vi "Keysight 34401A Cancellation Logic.vi"(8 "error in (no error)":errorcluster, 9 "session information":T1, 10 "measurement complete":refnum<user-event>, 11 "MeasurementContext in":refnum<class "MeasurementContext.lvclass">) -> (0 "error out":errorcluster, 3 "MeasurementContext out":refnum<class "MeasurementContext.lvclass">)   [LabVIEW 2020, in "Keysight 34401A DMM Measurement.lvlib"]
uses:
  Keysight 34401A DMM Measurement.lvlib
  <instrlib>/Agilent 34401/Agilent 34401.lvlib
  <vilib>/MeasurementLink/MeasurementLink Session Management Client/RPC Messages/ni_measurementlink_sessionmanagement_v1_ChannelMapping.ctl
  <vilib>/MeasurementLink/MeasurementLink Session Management Client/MeasurementLink Session Management Client.lvlib
  <vilib>/MeasurementLink/MeasurementLink Session Management Client/RPC Messages/nidevice_grpc_Session.ctl
  <vilib>/MeasurementLink/MeasurementLink Session Management Client/RPC Messages/ni_measurementlink_sessionmanagement_v1_SessionInformation.ctl
  <vilib>/MeasurementLink/MeasurementLink Measurement Server/Classes/MeasurementContext/MeasurementContext.lvclass
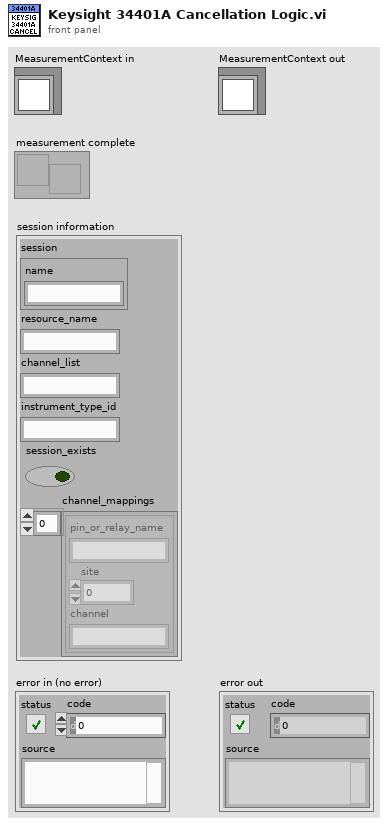
[diagram p1: front panel]
types:
  T1 = typedef "MeasurementLink Session Management Client.lvlib/ni_measurementlink_sessionmanagement_v1_SessionInformation.ctl" = cluster{"session":T2, "resource_name":string, "channel_list":string, "instrument_type_id":string, "session_exists":bool, "channel_mappings":T3[]}
  T2 = typedef "MeasurementLink Session Management Client.lvlib/nidevice_grpc_Session.ctl" = cluster{"name":string}
  T3 = typedef "MeasurementLink Session Management Client.lvlib/ni_measurementlink_sessionmanagement_v1_ChannelMapping.ctl" = cluster{"pin_or_relay_name":string, "site":i32, "channel":string}
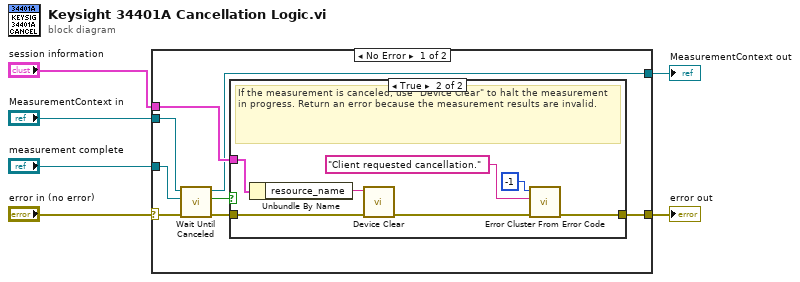
[diagram p0: block diagram]
diagram:
  n1 = case shown="No Error" "error in (no error)" {
    selector: "error in (no error)" -> [w7 w23]
    tunnel: "measurement complete" -> [w14 _]
    tunnel: "session information" -> [w13 _]
    tunnel: [w12 w23] -> w4
    tunnel: [w9 w24] -> w3
    tunnel: "MeasurementContext in" -> [w8 w24]
    frame No Error {
      n2 = call "Wait Until Canceled.vi"("error in (no error)"=w7, "measurement complete"=w14, "MeasurementContext in"=w8) -> ("error out"=w11:errorcluster, "is canceled?"=w10:bool, "MeasurementContext out"=w9:refnum<class "MeasurementContext.lvclass">)  [unwired: 6 in]
      n3 = case shown="True" w10 {
        tunnel: w11 -> [w15 w22]
        tunnel: [w15 w18] -> w12
        tunnel: w13 -> [_ w20]
        frame False {
        }
        frame True {
          # "If the measurement is canceled, use \"Device Clear\" to halt the measurement in progress. Return an error because the measurement results are invalid."
          n4 = Unbundle By Name(w20) -> ("resource_name"=w19:string)
          n5 = call <instrlib>:"Device Clear.vi"("error in (no error)"=w22, "VISA Resource Name"=w19) -> ("error out"=w21:errorcluster)  [unwired: 8 in, 1 out]
          n6 = call <vilib>:"Error Cluster From Error Code.vi"("error in (no error)"=w21, "error message (\"\")"="Client requested cancellation." ("error message (\"\")"), "error code (0)"=-1) -> ("error out"=w18:errorcluster)  [unwired: 6 in]
        }
      }
    }
    frame Error {
    }
  }
  "error out" <- w4
  "MeasurementContext out" <- w3
